vi "Process URLPatternInit.vi"(8 "error in (no error)":errorcluster, 9 "URL Pattern":T1, 10 "Type":string, 11 "Init":refnum<class "URLPattern.lvclass">) -> (0 "error out":errorcluster, 3 "Result":refnum<class "URLPattern.lvclass">)   [LabVIEW 2020, in "Stream.lvlib" / "URLPattern.lvclass"]
uses:
  URLPattern.lvclass
  URL Pattern Init.ctl
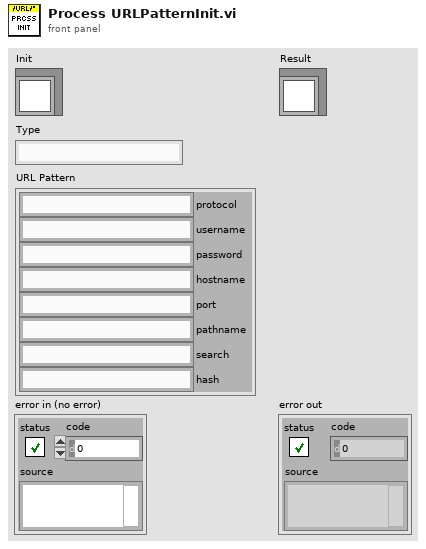
[diagram p1: front panel]
types:
  T1 = typedef "Stream.lvlib/URLPattern.lvclass/URL Pattern Init.ctl" = cluster{"protocol":string, "username":string, "password":string, "hostname":string, "port":string, "pathname":string, "search":string, "hash":string}
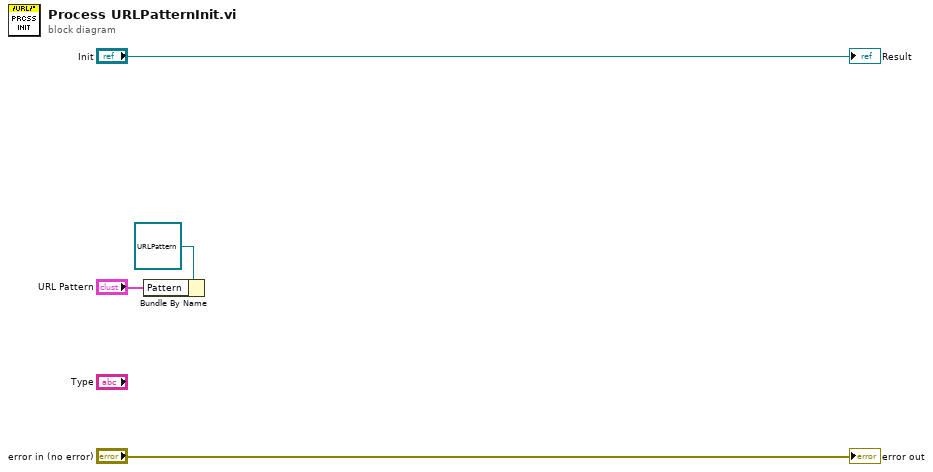
[diagram p0: block diagram]
diagram:
  n1 = Bundle By Name(cluster=refnum<class "URLPattern.lvclass"> refnum ("Stream:URLPattern.lvclass"), "Pattern"="URL Pattern") -> ()  [unwired: 1 out]
  "error out" <- "error in (no error)"
  "Result" <- "Init"
